vi "PM100D_Initialize.vi"() -> (0 "error out":errorcluster, 1 "Instrument":string, 2 "VISA out":refnum<visa-resource-name>, 4 "SN":string)   [LabVIEW 2011]
doc: "This VI scans for connected devices, that can be selected in a dialog box. Next steps\n- setting timeout\n- performing identification query\n- configuring the operation register to '512'; flag gets to HI when a new measurement value is ready to fetch\n- clear operation register"
uses:
  <vilib>/Instr/_visa.llb/VISA Find Search Mode.ctl
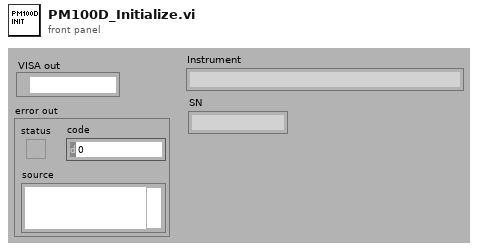
[diagram p1: front panel]
types:
  T1 = typedef "VISA Find Search Mode.ctl" = u32
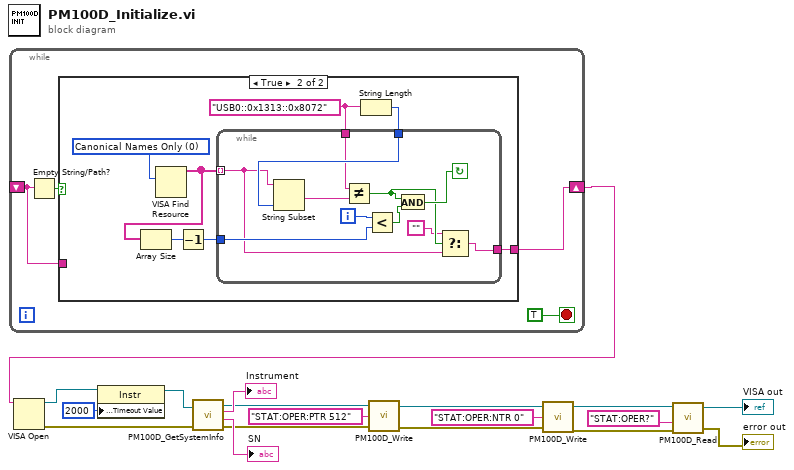
[diagram p0: block diagram]
diagram:
  n1 = while {
    shift-right: [w22] -> w1
    shift-left: _ -> [w20]
    stop <- TRUE stop-if-true
    n2 = Empty String/Path?(string/path=w20) -> (empty?=w21:bool)
    n3 = case shown="True" w21 {
      tunnel: [w23 w24] -> w22
      tunnel: w20 -> [w23 _]
      frame False {
      }
      frame True {
        w30 = T1 0 items=["Canonical Names Only"=0, "Aliases Only"=1, "Include Matching Aliases"=2, "Include All Aliases"=4] ("Search Mode")
        w28 = "USB0::0x1313::0x8072" ("element")
        n4 = VISA Find Resource(10:w30) -> (3:w27:string[])  [unwired: 1 in, 3 out]
        n5 = Array Size(array=w27) -> (size(s)=w26:i32)
        n6 = Decrement(x=w26) -> (x-1=w25:i32)
        n7 = String Length(string=w28) -> (length=w29:i32)
        n8 = while {
          tunnel: w29 -> [w41]
          tunnel: w27 -> [w32] mode=indexing
          tunnel: w28 -> [w40]
          tunnel: w25 -> [w37]
          tunnel: [w34] -> w24
          i -> [w38]
          stop <- w35 continue-if-true
          n9 = String Subset(string=w32, length (rest)=w41) -> (substring=w39:string)  [unwired: 1 in]
          n10 = Not Equal?(x=w40, y=w39) -> (x != y?=w33:bool)
          n11 = Less?(x=w38, y=w37) -> (x < y?=w36:bool)
          n12 = And(x=w33, y=w36) -> (x .and. y?=w35:bool)
          n13 = Select(t="", s=w33, f=w32) -> (s? t:f=w34:string)
        }
      }
    }
  }
  n14 = VISA Open(VISA resource name=w1) -> (VISA resource name=w14:refnum<visa-resource-name>, error out=w18:errorcluster)  [unwired: 1 in, 3 out]
  n15 = property class="Instr"(reference=w14, "General Settings:Timeout Value"=u32 2000) -> (reference out=w13:refnum<visa-resource-name>)  [unwired: 1 in, 1 out]
  n16 = call "PM100D_GetSystemInfo.vi"("VISA in"=w13, "error in"=w18) -> ("VISA out"=w11:refnum<visa-resource-name>, "Instrument"=→"Instrument":string, "SN"=→"SN":string, "error out"=w9:errorcluster)
  n17 = call "PM100D_Write.vi"("error in (no error)"=w9, "Command"="STAT:OPER:PTR 512", "VISA in"=w11) -> ("error out"=w8:errorcluster, "VISA out"=w10:refnum<visa-resource-name>)
  n18 = call "PM100D_Write.vi"("error in (no error)"=w8, "Command"="STAT:OPER:NTR 0", "VISA in"=w10) -> ("error out"=w2:errorcluster, "VISA out"=w6:refnum<visa-resource-name>)
  n19 = call "PM100D_Read.vi"("error in (no error)"=w2, "Command"="STAT:OPER?", "VISA in"=w6) -> ("error out"=→"error out":errorcluster, "VISA out"=→"VISA out":refnum<visa-resource-name>)  [unwired: 2 out]
